vi "ClusterToArray.vi"(0 "SensorData":T1={"cRIO Data"={"HallEffect Right (cm)"=0.0, "HallEffect Left (cm)"=0.0, "Optical Sensor 1 (V)"=0.0, "Optical Sensor 2 (V)"=0.0, "24V Voltage  (V)"=0.0, "24V Current (A)"=0.0, "Contactor H1 Continuity"=0.0, "Contactor L1 Continuity "=0.0, "Contactor H2 Continuity"=0.0, "Contactor L2 Continuity "=0.0, "Time (ms)"=0.0, "Displacement (ft)"=0.0, "Velocity (ft/s)"=0.0, "ABS Pressure 1 (psig)"=0.0, "ABS Pressure 2 (psig) "=0.0, "24 Temp Thermistor 1 (C)"=0.0, "24 Temp Thermistor 2 (C) "=0.0, "24 Temp Thermistor  3 (C) "=0.0, "24 Temp Thermistor 4 (C) "=0.0, "Brake PT(psig)"=0.0, "Tank PT(psig) "=0.0, "Pump PT(psig)"=0.0, "24 Temp Average(C) "=0.0, "High Voltage 1"=FALSE}, "IMU Data"={"x acceleration (g)"=0.0, "Pressure (psia)"=0.0, "Temperature (F)"=0.0}, "BMS Data"={"Max Cell Voltage (V)"=0.0, "Max Cell ID"=0.0, "Min Cell Voltage (V)"=0.0, "Min Cell ID"=0.0, "State of Charge (%)"=0.0, "Average Voltage (V)"=0.0, "Voltage Delta (V)"=0.0, "Pack Current (A)"=0.0, "Pack Voltage (V)"=0.0, "Max Resistance (Ohm)"=0.0, "Min Resistance (Ohm)"=0.0, "Average Resistance (Ohm)"=0.0, "Delta Resistance (Ohm)"=0.0, "Highest Temperature(F)"=0.0, "BmsStatus"={"isFault"=FALSE, "isolationMonitoring"=FALSE}}, "Motor Data"={" Velocity (RPM)"=0.0, " MotorTemp(C)"=0.0, " ControlTemp(C)"=0.0, " DcLinkVolt(V)"=0.0, " ErrorCode"=0.0, "IsAlive"=FALSE, "motorStatus"={"isReady"=FALSE, "isOn"=FALSE, "isOperEn"=FALSE, "isFault"=FALSE, "isVoltEn"=FALSE, "targetReached"=FALSE, "isWarning"=FALSE}, "motorControllerState"=1}} {"Motor Data"."motorControllerState" items=["unknown"=1, "boot-up"=0, "stopped"=4, "operational"=5, "pre-operational"=127, "connection lost"=128]}) -> (7 "Array":dbl[](array[numeric]))   [LabVIEW 2018]
uses:
  Type_Def/Type_Def Master_DataControl.ctl
  Type_Def/TypeDef_cRIOData.ctl
  Type_Def/Type_Def IMUData.ctl
  Type_Def/TypeDef_BMSData.ctl
  Type_Def/TypeDef_BmsStatus.ctl
  Type_Def/TypeDef FixedMotorData.ctl
types:
  T1 = typedef "Type_Def Master_DataControl.ctl" = cluster{"cRIO Data":T2, "IMU Data":T3, "BMS Data":T4, "Motor Data":T6}
  T2 = typedef "TypeDef_cRIOData.ctl" = cluster{"HallEffect Right (cm)":dbl, "HallEffect Left (cm)":dbl, "Optical Sensor 1 (V)":dbl, "Optical Sensor 2 (V)":dbl, "24V Voltage  (V)":dbl, "24V Current (A)":dbl, "Contactor H1 Continuity":dbl, "Contactor L1 Continuity ":dbl, "Contactor H2 Continuity":dbl, "Contactor L2 Continuity ":dbl, "Time (ms)":dbl, "Displacement (ft)":dbl, "Velocity (ft/s)":dbl, "ABS Pressure 1 (psig)":dbl, "ABS Pressure 2 (psig) ":dbl, "24 Temp Thermistor 1 (C)":dbl, "24 Temp Thermistor 2 (C) ":dbl, "24 Temp Thermistor  3 (C) ":dbl, "24 Temp Thermistor 4 (C) ":dbl, "Brake PT(psig)":dbl, "Tank PT(psig) ":dbl, "Pump PT(psig)":dbl, "24 Temp Average(C) ":dbl, "High Voltage 1":bool}
  T3 = typedef "Type_Def IMUData.ctl" = cluster{"x acceleration (g)":dbl, "Pressure (psia)":dbl, "Temperature (F)":dbl}
  T4 = typedef "TypeDef_BMSData.ctl" = cluster{"Max Cell Voltage (V)":dbl, "Max Cell ID":dbl, "Min Cell Voltage (V)":dbl, "Min Cell ID":dbl, "State of Charge (%)":dbl, "Average Voltage (V)":dbl, "Voltage Delta (V)":dbl, "Pack Current (A)":dbl, "Pack Voltage (V)":dbl, "Max Resistance (Ohm)":dbl, "Min Resistance (Ohm)":dbl, "Average Resistance (Ohm)":dbl, "Delta Resistance (Ohm)":dbl, "Highest Temperature(F)":dbl, "BmsStatus":T5}
  T5 = typedef "TypeDef_BmsStatus.ctl" = cluster{"isFault":bool, "isolationMonitoring":bool}
  T6 = typedef "TypeDef FixedMotorData.ctl" = cluster{" Velocity (RPM)":dbl, " MotorTemp(C)":dbl, " ControlTemp(C)":dbl, " DcLinkVolt(V)":dbl, " ErrorCode":dbl, "IsAlive":bool, "motorStatus":cluster{"isReady":bool, "isOn":bool, "isOperEn":bool, "isFault":bool, "isVoltEn":bool, "targetReached":bool, "isWarning":bool}, "motorControllerState":u16}
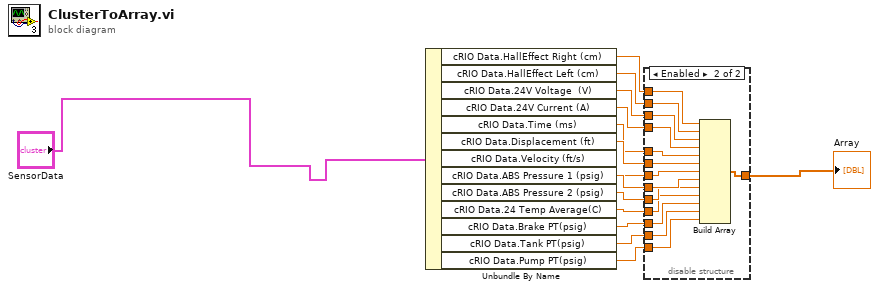
[diagram p0: block diagram]
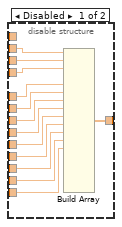
[diagram p2: hidden frame]
diagram:
  n1 = Unbundle By Name("SensorData") -> ("cRIO Data.HallEffect Right (cm)"=w2:dbl, "cRIO Data.HallEffect Left (cm)"=w3:dbl, "cRIO Data.24V Voltage  (V)"=w4:dbl, "cRIO Data.24V Current (A)"=w5:dbl, "cRIO Data.Time (ms)"=w6:dbl, "cRIO Data.Displacement (ft)"=w7:dbl, "cRIO Data.Velocity (ft/s)"=w8:dbl, "cRIO Data.ABS Pressure 1 (psig)"=w9:dbl, "cRIO Data.ABS Pressure 2 (psig)"=w10:dbl, "cRIO Data.24 Temp Average(C)"=w11:dbl, "cRIO Data.Brake PT(psig)"=w12:dbl, "cRIO Data.Tank PT(psig)"=w13:dbl, "cRIO Data.Pump PT(psig)"=w14:dbl)
  n2 = disable-structure shown="Enabled" {
    disable-tunnel: w3 -> [w34 w48]
    disable-tunnel: w4 -> [w33 w47]
    disable-tunnel: w5 -> [w32 w46]
    disable-tunnel: w6 -> [w30 w45]
    disable-tunnel: w7 -> [w29 w44]
    disable-tunnel: w8 -> [w28 w43]
    disable-tunnel: w9 -> [w27 w42]
    disable-tunnel: w10 -> [w26 w41]
    disable-tunnel: w11 -> [w25 w40]
    disable-tunnel: w12 -> [w24 w39]
    disable-tunnel: w13 -> [w23 w38]
    disable-tunnel: w14 -> [w22 w37]
    disable-tunnel: [w21 w36] -> w15
    disable-tunnel: w2 -> [_ w35]
    frame Disabled {
      n3 = Build Array(w34, w33, w32, w30, w29, w28, w27, w26, w25, w24, w23, w22) -> (w21:dbl[], w31:dbl, w20:dbl, w19:dbl, w18:dbl, w17:dbl, w16:dbl)
    }
    frame Enabled {
      n4 = Build Array(w35, w48, w47, w46, w45, w44, w43, w42, w41, w40, w39, w38, w37) -> (w36:dbl[])
    }
  }
  "Array" <- w15
